vi "CameraGlobals.vi"() -> ()   [LabVIEW 2024]
uses:
  <userlib>/ImageProcessing/QTLIB_2595_LV86/QT_Ref.ctl
panel:
  out "QT Ref":T1
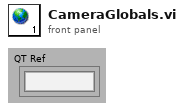
[diagram p1: front panel]
types:
  T1 = typedef "QT_Ref.ctl" = refnum<k1>
diagram:
